vi "Clear PDP Sticky Fault.vi"   [LabVIEW 2017]
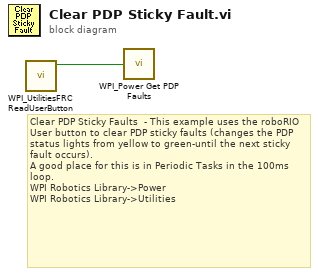
[diagram p0: block diagram]
diagram:
  # "Clear PDP Sticky Faults  - This example uses the roboRIO User button to clear PDP sticky faults (changes the PDP status lights from yellow to green-until the next sticky fault occurs). \nA good place for this is in Periodic Tasks in the 100ms loop. \nWPI Robotics Library->Power \nWPI Robotics Library->Utilities"
  n1 = call <vilib>:"WPI_UtilitiesFRC ReadUserButton.vi"() -> ("User Button"=w1:bool)  [unwired: 10 in, 1 out]
  n2 = call <vilib>:"WPI_Power Get PDP Faults.vi"("Clear Sticky Faults"=w1) -> ()  [unwired: 10 in, 5 out]
